vi "GT Arc YZC Override2WN.vi"(0 "cardNum":i16, 1 "crd":i16, 2 "y":i32, 3 "z":i32, 4 "yCenter":dbl, 5 "zCenter":dbl, 6 "circleDir":i16, 7 "error in (no error)":errorcluster caption="错误输入（无错误）", 8 "synVel":dbl, 9 "synAcc":dbl, 10 "velEnd":dbl, 11 "segNum":i32, 12 "fifo":i16) -> (20 "function return":i16, 27 "error out":errorcluster caption="错误输出")   [LabVIEW 2014, in "gts.lvlib"]
doc: "GT_API GT_ArcYZCOverride2WN(short cardNum,short crd,long y,long z,double yCenter,double zCenter,short circleDir,double synVel,double synAcc,double velEnd=0,long segNum=0,short fifo=0);"
uses:
  gts.lvlib
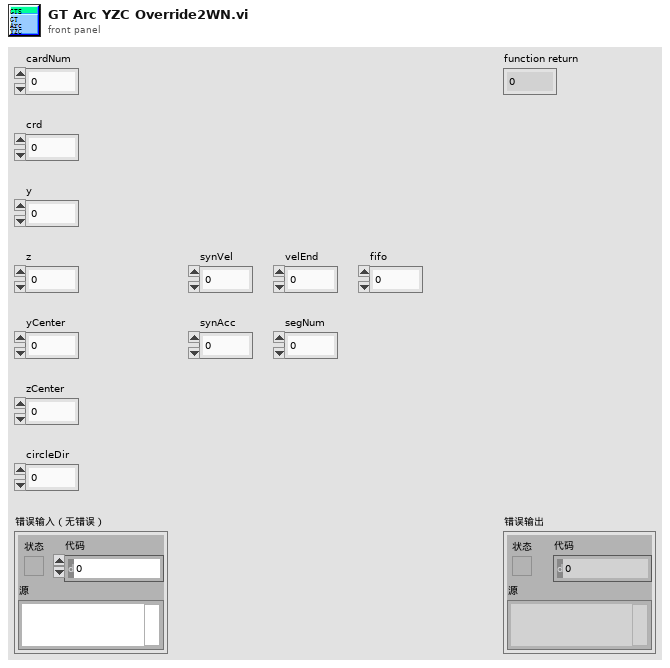
[diagram p1: front panel]
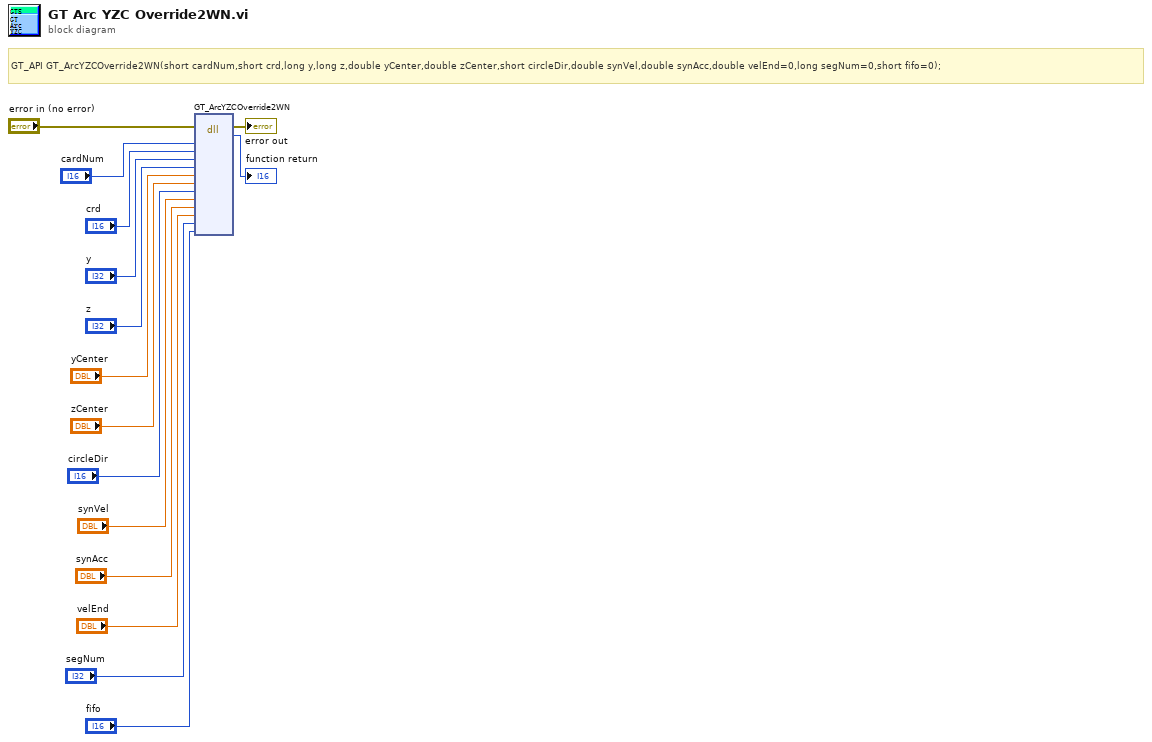
[diagram p0: block diagram]
diagram:
  # "GT_API GT_ArcYZCOverride2WN(short cardNum,short crd,long y,long z,double yCenter,double zCenter,short circleDir,double synVel,double synAcc,double velEnd=0,long segNum=0,short fifo=0);"
  n1 = dll-call lib="PTH2habs D固高科技资料GTS控制卡GTS卡18年上半年资料dllVC32bit\nmulti_cardgts.*" fn="GT_ArcYZCOverride2WN"(error in="error in (no error)", "cardNum"="cardNum", "crd"="crd", "y"="y", "z"="z", "yCenter"="yCenter", "zCenter"="zCenter", "circleDir"="circleDir", "synVel"="synVel", "synAcc"="synAcc", "velEnd"="velEnd", "segNum"="segNum", "fifo"="fifo") -> (error out=→"error out":errorcluster, →"function return":i16)  [unwired: 14 in, 1 out]
